vi "stringArrayToEnum.vi"() -> ()   [LabVIEW 2013]
panel:
  out "Ringtext.Text":string
  in  "Enum":enum16{"This", "is", "after"}(ring)
  in  "Ring":u16(ring) items=["enum 0", "enum 1", "enum 2"]
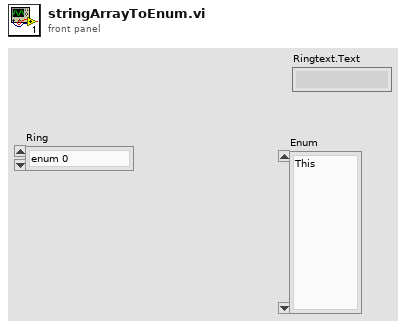
[diagram p1: front panel]
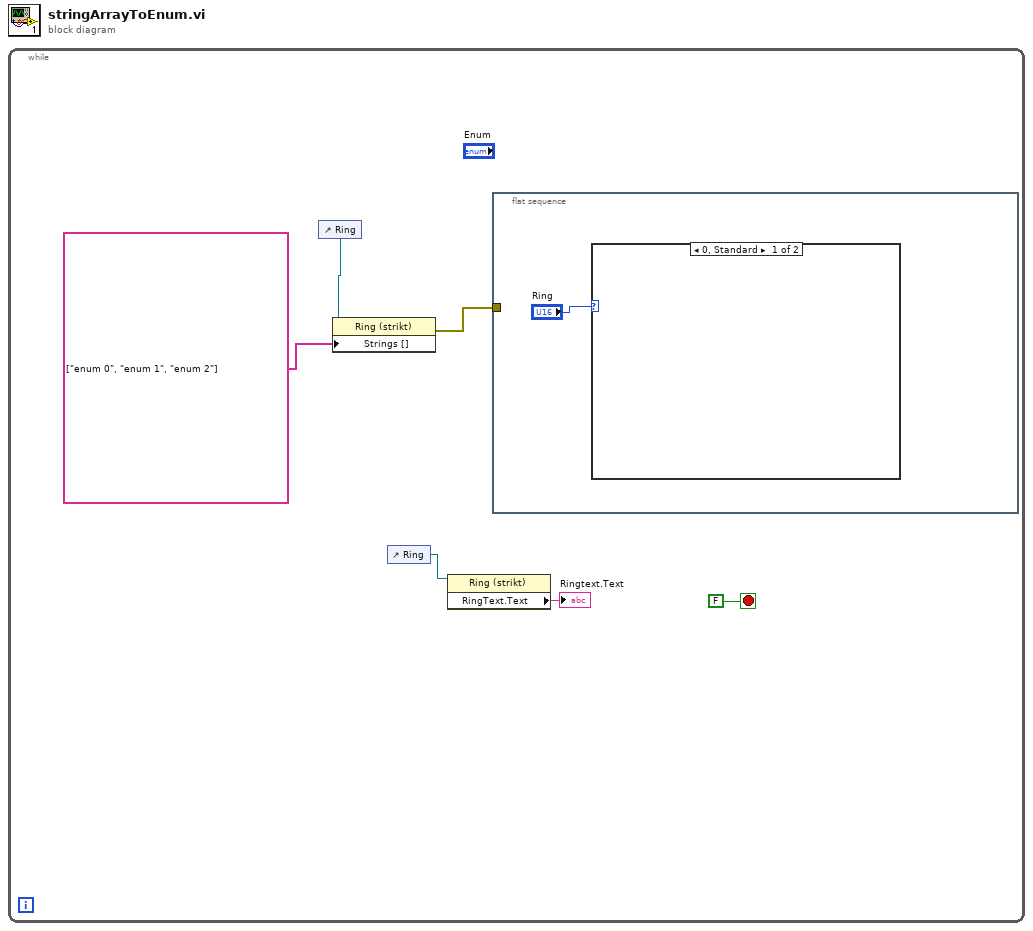
[diagram p0: block diagram]
diagram:
  n1 = while {
    stop <- FALSE stop-if-true
    n2 = control-ref of="Ring"() -> (w6:refnum<vi>)
    n3 = property class="Ring (strikt)"(reference=w6, "Strings []"=string[] ["enum 0", "enum 1", "enum 2"]) -> (error out=w5:errorcluster)  [unwired: 1 in, 1 out]
    n4 = control-ref of="Ring"() -> (w2:refnum<vi>)
    n5 = property class="Ring (strikt)"(reference=w2) -> ("RingText.Text"=→"Ringtext.Text":string)  [unwired: 1 in, 2 out]
    n6 = flat-sequence {
      tunnel: w5 -> [_]
      frame #0 {
        n7 = case shown="0, Standard" "Ring" {
          frame 0, Default {
          }
          frame 1 {
          }
        }
      }
    }
  }
